vi "String.Remove Quotes.vi"(11 "String With Quotes":string) -> (2 "Quotes Removed":bool, 3 "String No Quotes":string)   [LabVIEW 2024, in "EQMF.lvlib" / "String Utils.lvlib"]
uses:
  String Utils.lvlib
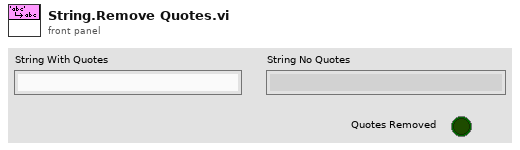
[diagram p1: front panel]
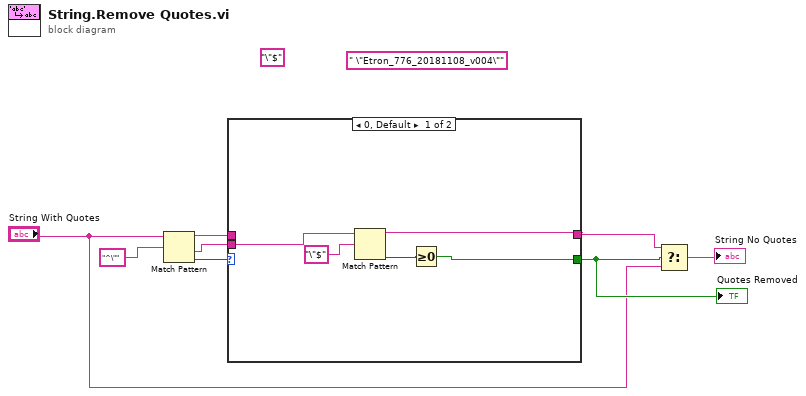
[diagram p0: block diagram]
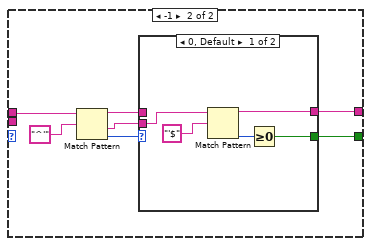
[diagram p2: hidden frame]
diagram:
  (unwired) "\"$" ("regular expression")
  (unwired) " \"Etron_776_20181108_v004\""
  n1 = Match Pattern(string="String With Quotes", regular expression="^\"") -> (before substring=w5:string, after substring=w6:string, offset past match=w7:i32)  [unwired: 1 in, 1 out]
  n2 = case shown="0, Default" w7 {
    tunnel: w6 -> [w12 _]
    tunnel: w5 -> [_ w19]
    tunnel: [w10 w15] -> w3
    tunnel: [w9 w14] -> w4
    frame 0, Default {
      n3 = Match Pattern(string=w12, regular expression="\"$") -> (before substring=w10:string, offset past match=w11:i32)  [unwired: 1 in, 2 out]
      n4 = Greater Or Equal To 0?(x=w11) -> (x >= 0?=w9:bool)
    }
    frame -1 {
      n5 = Match Pattern(string=w19, regular expression="^'") -> (before substring=w17:string, after substring=w16:string, offset past match=w18:i32)  [unwired: 1 in, 1 out]
      n6 = case shown="0, Default" w18 {
        tunnel: w17 -> [_ _]
        tunnel: w16 -> [w24 _]
        tunnel: [w21 _] -> w15
        tunnel: [w22 _] -> w14
        frame 0, Default {
          n7 = Match Pattern(string=w24, regular expression="'$") -> (before substring=w21:string, offset past match=w23:i32)  [unwired: 1 in, 2 out]
          n8 = Greater Or Equal To 0?(x=w23) -> (x >= 0?=w22:bool)
        }
        frame -1 {
        }
      }
    }
  }
  "Quotes Removed" <- w4
  n9 = Select(t=w3, s=w4, f="String With Quotes") -> (s? t:f=→"String No Quotes":string)
